vi "CMI ckd2 Set Divider Rate.vi"(8 "error in":errorcluster, 10 "clock rate [Hz]":dbl=1000.0, 11 "session":T1) -> (0 "error out":errorcluster, 2 "clock rate out [Hz]":dbl format="%#_8p", 3 "session out":T1)   [LabVIEW 2013, in "AWG.lvlib"]
doc: "Sets division factor to main channel so it outputs desired frequency.\nDepending on the setting of reference clock source it either uses measured input clock rate or manually entered input clock rate as a reference. Note the meter has measurement latency at least 1 second or so."
uses:
  AWG.lvlib
  CMI ckd2 Session.ctl
  CMI ckd2 Source Mode.ctl
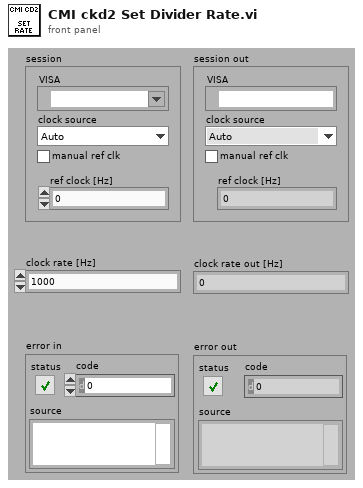
[diagram p1: front panel]
types:
  T1 = typedef "AWG.lvlib/CMI ckd2 Session.ctl" = cluster{"VISA":refnum<visa-resource-name>, "clock source":T2, "manual ref clk":bool, "ref clock [Hz]":dbl}
  T2 = typedef "AWG.lvlib/CMI ckd2 Source Mode.ctl" = enum16{"Auto", "LF clock", "HF clock", "Internal"}
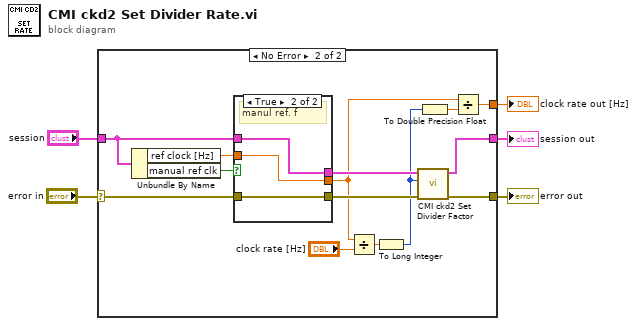
[diagram p0: block diagram]
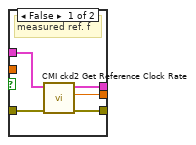
[diagram p3: hidden frame]
diagram:
  n1 = case shown="No Error" "error in" {
    selector: "error in" -> [w6 w21]
    tunnel: [w7 w12] -> w3
    tunnel: [w6 w13] -> w5
    tunnel: "session" -> [w7 w19]
    tunnel: [_ w8] -> w1
    frame Error {
    }
    frame No Error {
      n2 = Unbundle By Name(w19) -> ("ref clock [Hz]"=w18:dbl, "manual ref clk"=w20:bool)
      n3 = case shown="True" w20 {
        tunnel: w21 -> [w26 w27]
        tunnel: w19 -> [w25 w28]
        tunnel: [w24 w27] -> w17
        tunnel: [w23 w28] -> w16
        tunnel: [w22 w29] -> w11
        tunnel: w18 -> [_ w29]
        frame False {
          # "measured ref. f"
          n4 = call "CMI ckd2 Get Reference Clock Rate.vi"("error in"=w26, "session"=w25) -> ("error out"=w24:errorcluster, "clock rate [Hz]"=w22:dbl, "session out"=w23:T1)  [unwired: 7 in]
        }
        frame True {
          # "manul ref. f"
        }
      }
      n5 = Divide(x=w11, y="clock rate [Hz]") -> (x/y=w14:dbl)
      n6 = To Long Integer(number=w14) -> (32bit integer=w10:i32)
      n7 = call "CMI ckd2 Set Divider Factor.vi"("error in"=w17, "division factor (1)"=w10, "session"=w16) -> ("error out"=w13:errorcluster, "session out"=w12:T1)  [unwired: 7 in]
      n8 = To Double Precision Float(number=w10) -> (double precision float=w9:dbl)
      n9 = Divide(x=w11, y=w9) -> (x/y=w8:dbl)
    }
  }
  "error out" <- w5
  "session out" <- w3
  "clock rate out [Hz]" <- w1
